vi "send_scpi.vi"(9 "Host":string) -> ()   [LabVIEW 2014]
uses:
  <vilib>/Easy HTTP Client/Easy HTTP.lvlib
panel:
  out "Response":string
  in  "Slot":string
  in  "SCPI":string
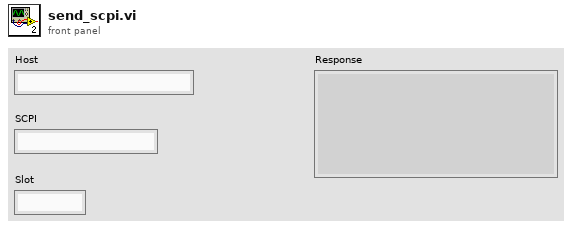
[diagram p1: front panel]
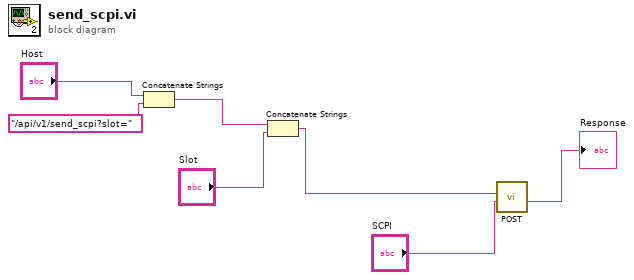
[diagram p0: block diagram]
diagram:
  n1 = Concatenate Strings("Host", "/api/v1/send_scpi?slot=") -> (w5:string)
  n2 = Concatenate Strings(w5, "Slot") -> (w2:string)
  n3 = call <vilib>:"POST.vi"("data"="SCPI", "url"=w2) -> ("body"=→"Response":string)  [unwired: 5 in, 4 out]
